vi "IT8800-Clear Protection Alarm.vi"(8 "error in":errorcluster, 11 "IT8800 Setting In In":T1={"VISA Resource Name"="", "Baud Rate"=19200, "Stop Bits"=20, "Wait For Read(ms)"=0} {"Stop Bits" items=["1.0"=10, "2.0"=20]; "Baud Rate" items=["2400"=2400, "4800"=4800, "9600"=9600, "19200"=19200]}) -> (0 "error out":errorcluster, 3 "IT8800 Setting In Out":T1={"VISA Resource Name"="", "Baud Rate"=19200, "Stop Bits"=20, "Wait For Read(ms)"=0} {"Stop Bits" items=["1.0"=10, "2.0"=20]; "Baud Rate" items=["2400"=2400, "4800"=4800, "9600"=9600, "19200"=19200]})   [LabVIEW 2018]
uses:
  Data Def/IT8800-Setting.ctl
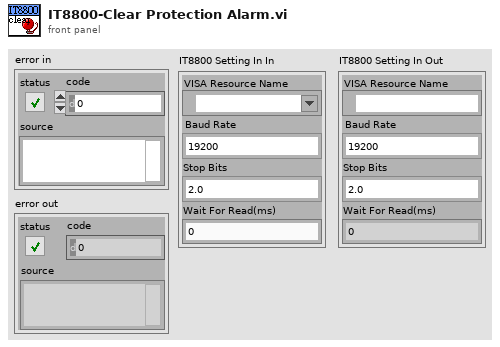
[diagram p1: front panel]
types:
  T1 = typedef "IT8800-Setting.ctl" = cluster{"VISA Resource Name":refnum<visa-resource-name>, "Baud Rate":u32, "Stop Bits":u16, "Wait For Read(ms)":u32}
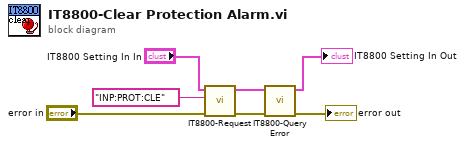
[diagram p0: block diagram]
diagram:
  n1 = call "IT8800-Request.vi"("error in"="error in", "Command"="INP:PROT:CLE" ("write buffer"), "IT8800 Setting In In"="IT8800 Setting In In") -> ("error out"=w6:errorcluster, "IT8800 Setting In Out"=w2:T1)  [unwired: 6 in, 1 out]
  n2 = call "IT8800-Query Error.vi"("error in"=w6, "IT8800 Setting In In"=w2) -> ("error out"=→"error out":errorcluster, "IT8800 Setting In Out"=→"IT8800 Setting In Out":T1)  [unwired: 8 in]
